vi "File_Get Valid Folder.vi"(8 "Error":errorcluster, 9 "Message":string="Select the Cal File Folder", 11 "File Folder":path) -> (0 "Error Out":errorcluster, 2 "Valid Out":bool, 3 "Folder Out":path)   [LabVIEW 2015]
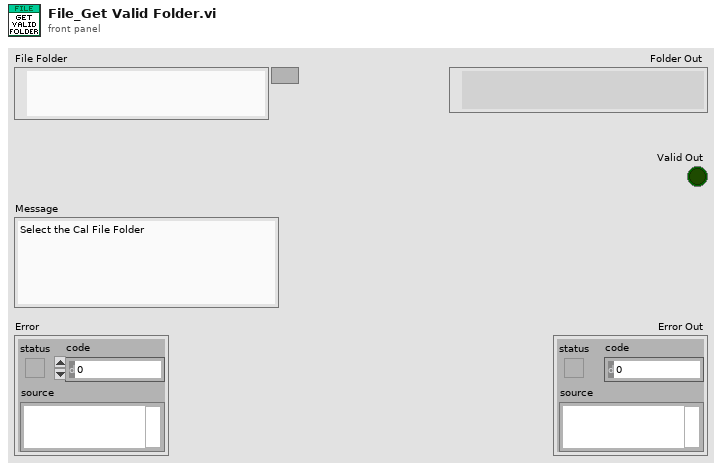
[diagram p1: front panel]
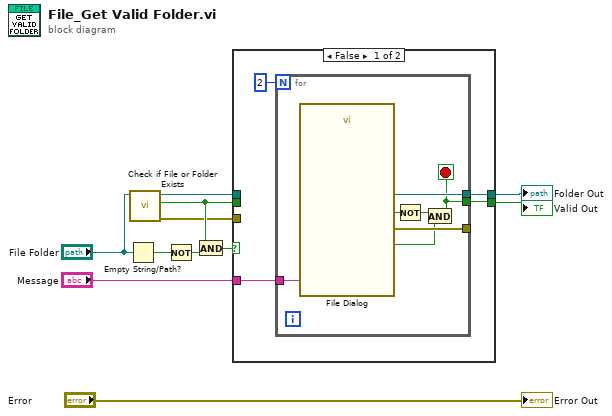
[diagram p0: block diagram]
diagram:
  n1 = Empty String/Path?(string/path="File Folder") -> (empty?=w10:bool)
  n2 = call <vilib>:"Check if File or Folder Exists.vi"("path"="File Folder") -> ("error out"=w2:errorcluster, "file or folder exists?"=w3:bool, "dup path"=w4:path)  [unwired: 8 in]
  n3 = Not(x=w10) -> (.not. x?=w11:bool)
  n4 = And(x=w3, y=w11) -> (x .and. y?=w8:bool)
  n5 = case shown="False" w8 {
    tunnel: "Message" -> [w15 _]
    tunnel: [w14 w24] -> w6
    tunnel: [w13 w23] -> w5
    tunnel: w4 -> [_ w24]
    tunnel: w3 -> [_ w23]
    tunnel: w2 -> [_ _]
    frame False {
      n6 = for {
        N: 2 -> [_]
        tunnel: w15 -> [w22]
        tunnel: [w20] -> w14
        tunnel: [w16] -> w13
        tunnel: [w21] -> _
        stop <- w16 stop-if-true
        n7 = call "File Dialog"("prompt"=w22) -> ("selected path"=w20:path, "exists"=w17:bool, "cancelled"=w19:bool, "error out"=w21:errorcluster)  [unwired: 11 in]
        n8 = Not(x=w19) -> (.not. x?=w18:bool)
        n9 = And(x=w18, y=w17) -> (x .and. y?=w16:bool)
      }
    }
    frame True {
    }
  }
  "Folder Out" <- w6
  "Valid Out" <- w5
  "Error Out" <- "Error"
